vi "Inject_Velocity_Ratio.vi"() -> (5 "Plug in titles":string[](array[string]), 7 "Plug in values":string[](array[string]))   [LabVIEW 2010]
uses:
  Globals/Meas_global.vi
  Globals/Extra_Commands_Global.vi
  ADAM Client/Sub VIs/ADAM Controls/Update_scan_value.ctl
panel:
  out "Uo/Ulocal":dbl
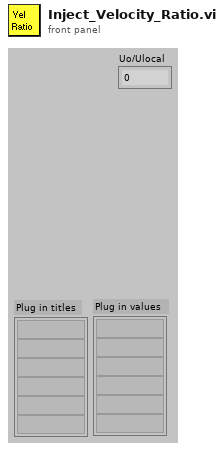
[diagram p1: front panel]
types:
  T1 = typedef "Velocity_cluster.ctl" = cluster{"Name":string, "U":dbl, "u^2":dbl, "u^3/(u^2)^(1.5)":dbl, "u^4/(u^2)^2 -3":dbl, "% u'/U":dbl, "Mean % Err":dbl, "u^4":dbl}
  T2 = typedef "Update_scan_value.ctl" = cluster{"Channel Name":string, "New Value":dbl}
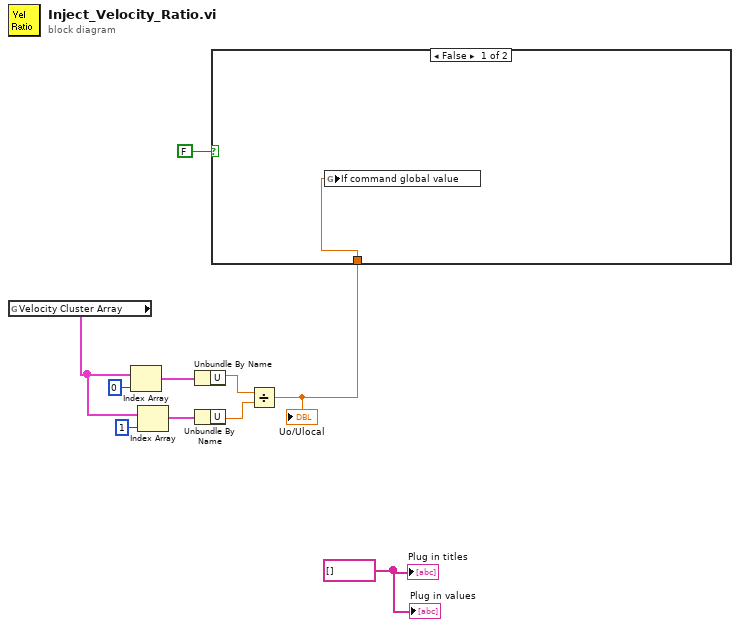
[diagram p0: block diagram]
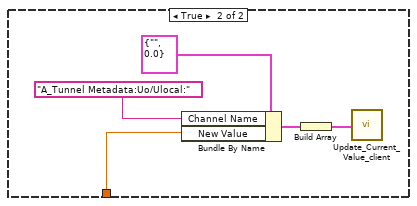
[diagram p2: hidden frame]
diagram:
  w10 = string[] [] ("Plug in titles")
  n1 = global read "Meas_global.vi" "Velocity Cluster Array"() -> (w4:T1[])
  n2 = Index Array(array=w4, index=0) -> (element=w5:T1)
  n3 = Index Array(array=w4, index=1) -> (element=w6:T1)
  n4 = Unbundle By Name(w5) -> ("U"=w8:dbl)
  n5 = Unbundle By Name(w6) -> ("U"=w7:dbl)
  n6 = Divide(x=w8, y=w7) -> (x/y=w9:dbl)
  "Uo/Ulocal" <- w9
  n7 = case shown="False" FALSE {
    tunnel: w9 -> [w11 w16]
    frame False {
      n8 = global write "Extra_Commands_Global.vi" "If command global value"(w11) -> ()
    }
    frame True {
      n9 = Bundle By Name(cluster=T2 {"Channel Name"="", "New Value"=0.0} ("Update Scan Value Cluster"), "Channel Name"="A_Tunnel Metadata:Uo/Ulocal:", "New Value"=w16) -> (w13:T2)
      n10 = Build Array(w13) -> (w14:T2[])
      n11 = call "Update_Current_Value_client.vi"("Update array in"=w14) -> ()  [unwired: 1 in]
    }
  }
  "Plug in values" <- w10
  "Plug in titles" <- w10
